vi "Initialize.vi"(8 "error in (no error)":errorcluster, 11 "FTPProtocol in":refnum<class "FTPProtocol.lvclass">) -> (0 "error out":errorcluster, 3 "FTPProtocol out":refnum<class "FTPProtocol.lvclass">)   [LabVIEW 2020, in "CSM-FileSync.lvlib" / "FTPProtocol.lvclass"]
uses:
  FTPProtocol.lvclass
  FTP Toolkit/FTP Class/FTP.lvclass
  FTPProtocol.lvclass/FTPProtocol.ctl
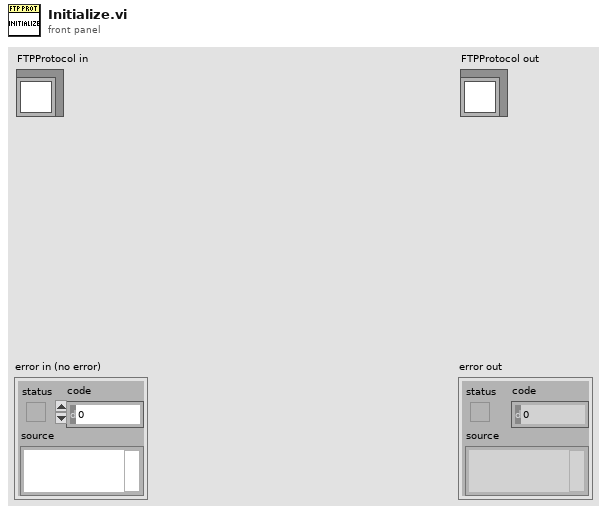
[diagram p1: front panel]
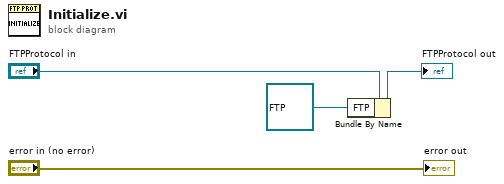
[diagram p0: block diagram]
diagram:
  n1 = Bundle By Name(cluster="FTPProtocol in", "FTP"=refnum<class "FTP.lvclass"> refnum) -> (→"FTPProtocol out":refnum<class "FTPProtocol.lvclass">)
  "error out" <- "error in (no error)"
